vi "MainLoop2.vi"() -> ()   [LabVIEW 2021] (continued)
                                                                                                                                                                                   256705543", "Inter-pellet_interval", "0", "201", "0", "0", "0"], ["15/06/2022", "17:54:17", "                                                                                                                                                                                                                                                                                                                                                                                                                                                                                                                                                                                                                                                                                                                                                                                                                                                                                                                                                                                                                                                                                                                                                                                                                                                                                                                                                                                                                                                                                                                                                                                                                                                                                                                                                                                                                                                                                                                                                                                                                                                                                                                                                                                                                                                                                                                                                                                                                                                                                                                                                                                                                                                                                                                                                                                                                                                                                                                                                                                                                                                                                                                                                                                                                                                                                                                                                                                                                                                                                                                                                                                                                                                                                                                                                                                                                                                                                                                                                                                                                                                                                                                                                                                                                                                                                                                                                                                                                                                                                                                                                                                                                                                                                                                                                                                                                                                                                                                                                                                                                                                                                                                                                                                                                                                                                                                                                                                                                                                                                                                                                                                                                                                                                                                                                                                                                                                                                                                                                                                                                                                                                                                                                                                                                                                                                                                                                                                                                                                                                                                                                                                                                                                                                                                                                                                                                                                                                                                                                                                                                                                                                                                                                                                                                                                                                                                                                                                                                                                                                                                                                                                                                                                                                                                                                                                                                                                                                                                                                                                                                                                                                                                                                                                                                                                                                                                                                                                                                                                                                                                                                                                                                                                                                                                                                                                                                                                                                                                                                                                                                                                                                                                                                                                                                                                                                                                                                                                                                                                                                                                                                                                                                                                                                                                                                                                                                                                                                                                                                                                                                                                                                                                                                                                                                                                                                                                                                                                                                                                                                                                                                                                                                                                                                                                                                                                                                                                                                                                                                                                                                                                                                                                                                                                                                                                                                                                                                                                                                                                                                                                                                                                                                                          256715699", "3 pellets delivered total", "0", "201", "0", "0", "0"], ["15/06/2022", "17:54:17", "                                                                                                                                                                                                                                                                                                                                                                                                                                                                                                                                                                                                                                                                                                                                                                                                                                                                                                                                                                                                                                                                                                                                                                                                                                                                                                                                                                                                                                                                                                                                                                                                                                                                                                                                                                                                                                                                                                                                                                                                                                                                                                                                                                                                                                                                                                                                                                                                                                                                                                                                                                                                                                                                                                                                                                                                                                                                                                                                                                                                                                                                                                                                                                                                                                                                                                                                                                                                                                                                                                                                                                                                                                                                                                                                                                                                                                                                                                                                                                                                                                                                                                                                                                                                                                                                                                                                                                                                                                                                                                                                                                                                                                                                                                                                                                                                                                                                                                                                                                                                                                                                                                                                                                                                                                                                                                                                                                                                                                                                                                                                                                                                                                                                                                                                                                                                                                                                                                                                                                                                                                                                                                                                                                                                                                                                                                                                                                                                                                                                                                                                                                                                                                                                                                                                                                                                                                                                                                                                                                                                                                                                                                                                                                                                                                                                                                                                                                                                                                                                                                                                                                                                                                                                                                                                                                                                                                                                                                                                                                                                                                                                                                                                                                                                                                                                                                                                                                                                                                                                                                                                                                                                                                                                                                                                                                                                                                                                                                                                                                                                                                                                                                                                                                                                                                                                                                                                                                                                                                                                                                                                                                                                                                                                                                                                                                                                                                                                                                                                                                                                                                                                                                                                                                                                                                                                                                                                                                                                                                                                                                                                                                                                                                                                                                                                                                                                                                                                                                                                                                                                                                                                                                                                                                                                                                                                                                                                                                                                                                                                                                                                                                                                                                                                                                                                                                                                                                                                                                                                                                                                                                                                                                                              256716167", "3 pellets delivered total", "0", "201", "3", "0", "0"], ["15/06/2022", "17:54:50", "256749394", "3 pellets delivered total", "0", "120", "0", "0", "0"], ["15/06/2022", "17:54:50", "256749419", "Condition: j - 120", "0", "120", "0", "0", "0"], ["15/06/2022", "17:54:52", "256750710", "Nest beam break", "0", "120", "0", "0", "0"], ["15/06/2022", "18:19:22", "                                                                                                                                                                                                                                                                                                                                                                                                                                                                                                                                                                                                                                                                                                                                                                                                                                                                                                                                                                                                                                                                                                                                                                                                                                                                                                                                                                                                                                                                                                                                                                                                                                                                                                                                                                                                                                                                                                                                                                                                                                                                                                                                                                                                                                                                                                                                                                                                                                                                                                                                                                                                                                                                                                                                                                                                                                                                                                                                                                                                                                                                                                                                                                                                                                                                                                                                                                                                                                                                                                                                                                                                                                                                                                                                                                                                                                                                                                                                                                                                                                                                                                                                                                                                                                                                                                                                                                                                                                                                                                                                                                                                                                                                                                                                                                                                                                                                                                                                                                                                                                                                                                                                                                                                                                                                                                                                                                                                                                                                                                                                                                                                                                                                                                                                                                                                                                                                                                                                                                                                                                                                                                                                                                                                                                                                                                                                                                                                                                                                                                                                                                                                                                                                                                                                                                                                                                                                                                                                                                                                                                                                                                                                                                                                                                                                                                                                                                                                                                                                                                                                                                                                                                                                                                                                                                                                                                                                                                                                                                                                                                                                                                                                                                                                                                                                                                                                                                                                                                                                                                                                                                                                                                                                                                                                                                                                                                                                                                                                                                                                                                                                                                                                                                                                                                                                                                                                                                                                                                                                                                                                                                                                                                                                                                                                                                                                                                                                                                                                                                                              258221447", "1469059 ms in nest", "1469059", "120", "0", "0", "0"]]
  in  "Save event file?":bool=TRUE
  in  "file path (dialog if empty)":path=path "C:/Data/av_maze/cohort1/mouseX_202206XXtxt"
  # "Social\n\nWater\n\nFood\n\nMiddle 1\n\nMiddle 2\n\nHome cage"
  # "Low (0)     Medium (1)    High(2)"
  # "Pellets \n\nWater drops\n\nSocial time (ms)"
  # "This should stay at 1"
  # "Social                Water                  Food               Middle            Middle 2       Home cage"
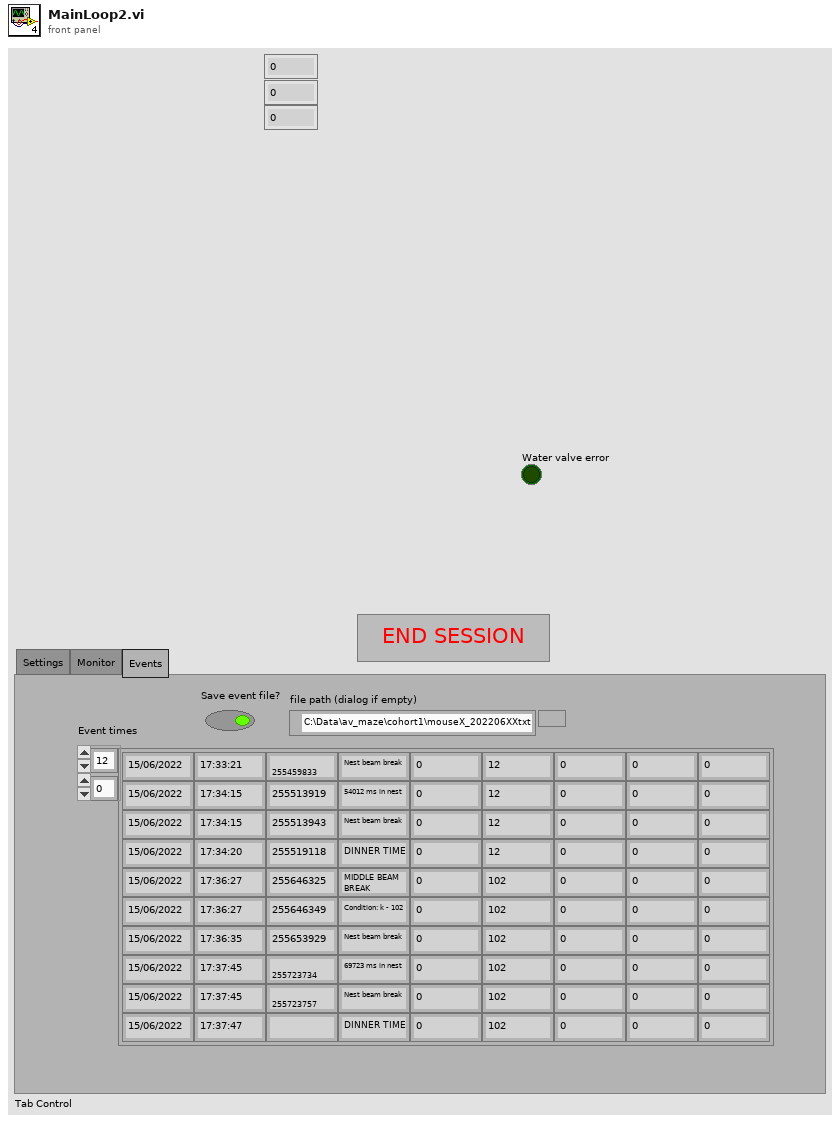
[diagram p1: front panel]
types:
  T1 = enum32{"All drives change and different", "One drive changes", "All drives same, but change"}
  T2 = typedef "XDNodeRunTimeDep.lvlib/timing_clust.ctl" = cluster{"Expected End [f-1]":u64, "Actual End [f-1]":u64, "Finished Late? [f-1]":bool, "Expected End [i-1]":u64, "Actual End [i-1]":u64, "Finished Late? [i-1]":bool, "Expected Start [i]":u64, "Actual Start [i]":u64, "Expected Start [f]":u64, "Actual Start [f]":u64, "Source Name":string, "Structure Name":string, "Period":i64, "Deadline":i64, "Offset":i64, "Start":i64, "Priority":i32, "Timeout":i32, "Mode":T3, "Wakeup Reason":T4, "Error":errorcluster, "Source Type":string, "Secondary Source Type":string, "Global End Time":u64, "Global Start Time":u64, "Frame Duration":u64, "Iteration Duration":u64, "Assigned CPU":i32, "I/O Scan Engine Mode":u32}
  T3 = typedef "XDNodeRunTimeDep.lvlib/nitl_modes.ctl" = enum32{"No Change", "Process missed periods, maintain original phase", "Discard missed periods, maintain original phase", "Process missed periods, ignore original phase", "Discard missed periods, ignore original phase"}
  T4 = typedef "XDNodeRunTimeDep.lvlib/wakeup.ctl" = enum32{"Normal", "Aborted", "Asynchronous wakeup", "Timing source error", "Timed loop error", "Timeout"}
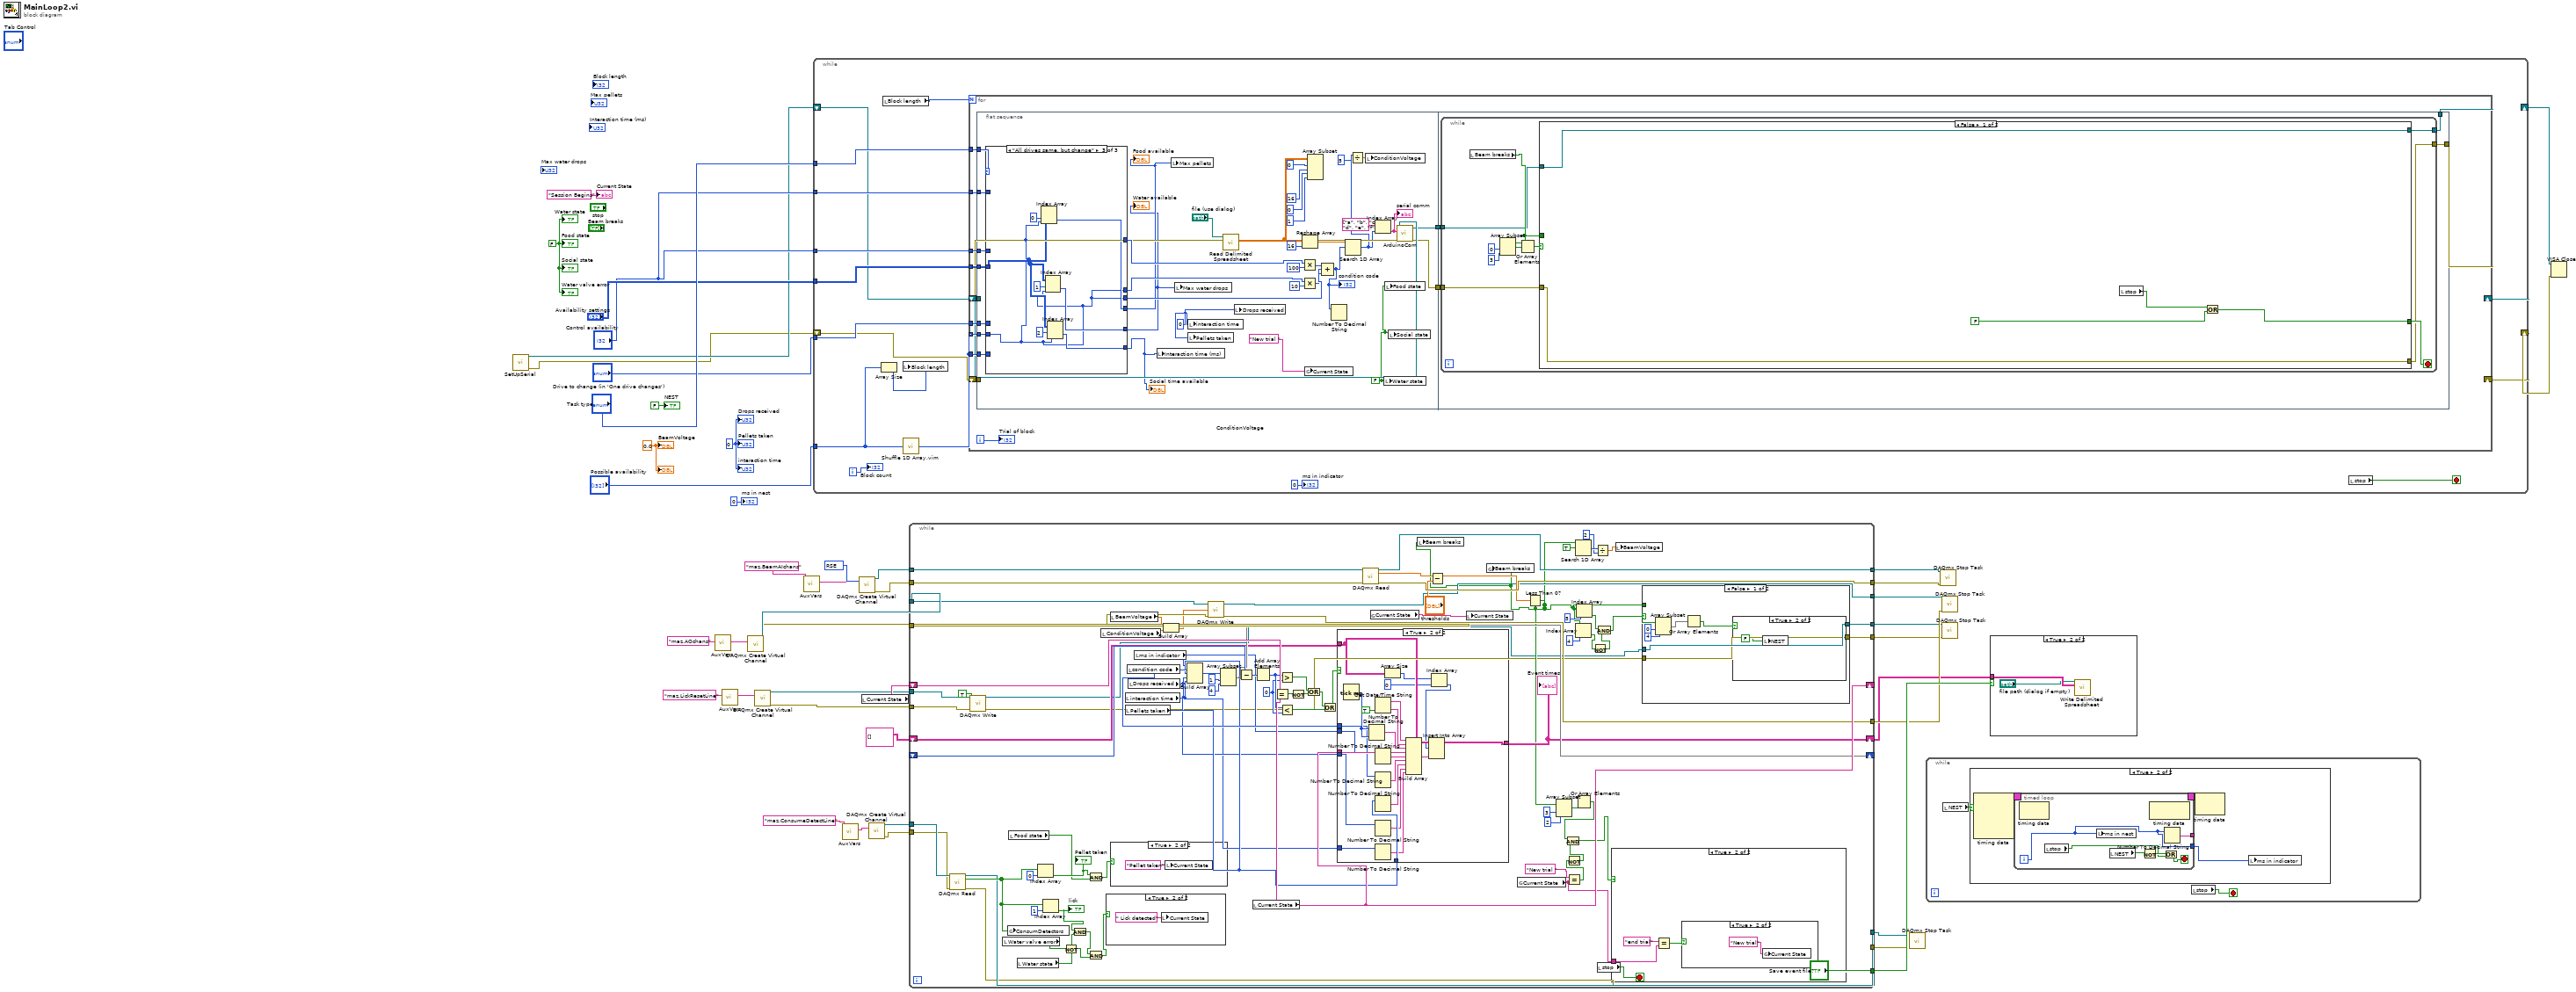
[diagram p0: block diagram]
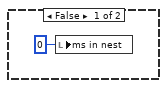
[diagram p2: hidden frame]
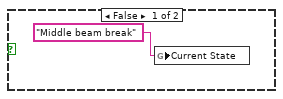
[diagram p7: hidden frame]
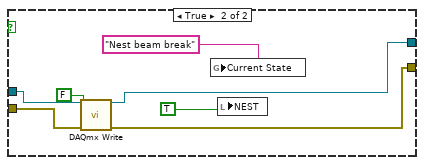
[diagram p9: hidden frame]
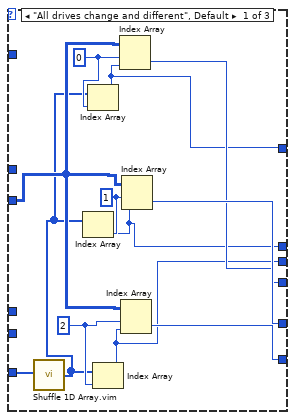
[diagram p11: hidden frame]
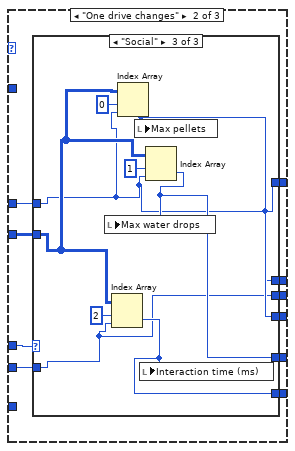
[diagram p12: hidden frame]
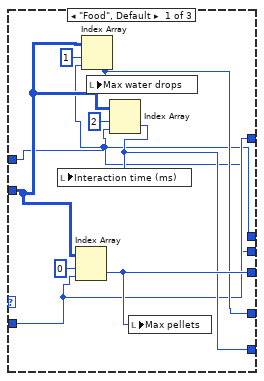
[diagram p13: hidden frame]
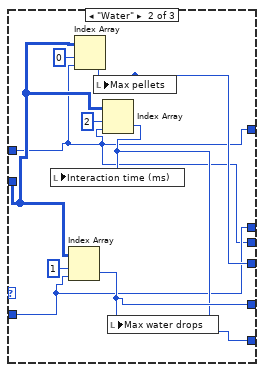
[diagram p14: hidden frame]
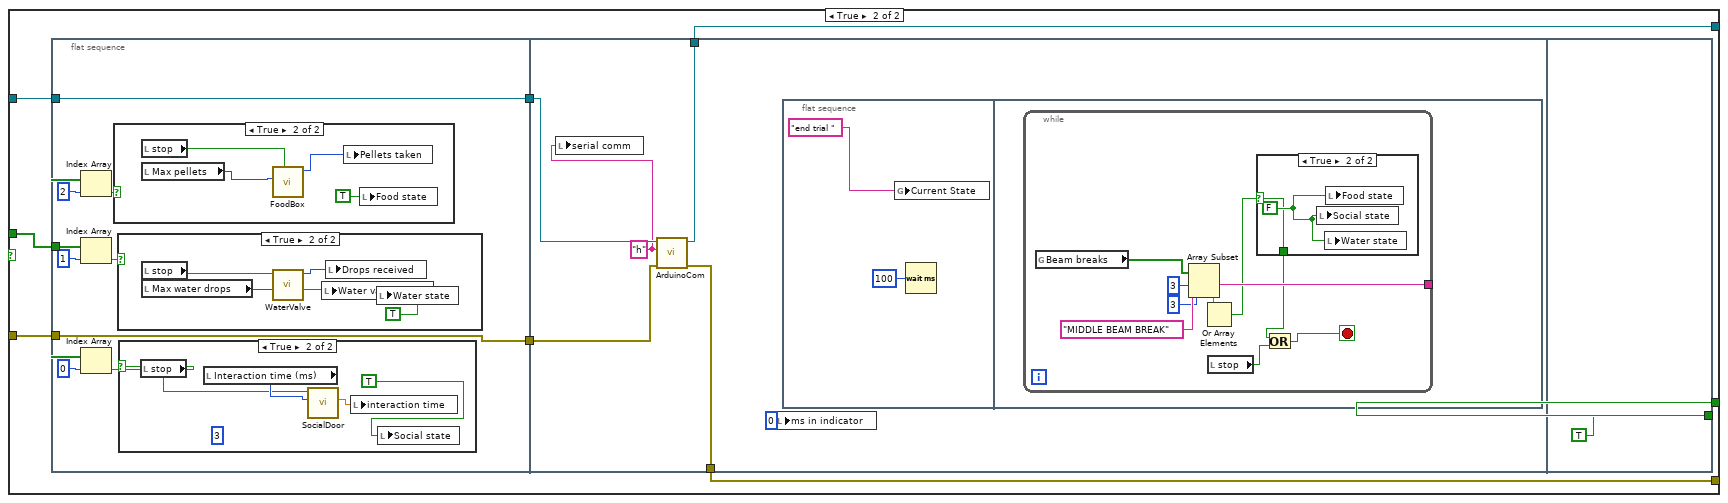
[diagram p15: hidden frame]
diagram:
  w7 = FALSE ("Water state")
  w16 = u32 0 ("Pellets taken")
  w27 = 0.0 ("BeamVoltage")
  w32 = 10083 items=["Default"=-1, "RSE"=10083, "NRSE"=10078, "Differential"=10106, "Pseudodifferential"=12529] ("input terminal configuration")
  n1 = call "SetUpSerial.vi"() -> ("error out"=w19:errorcluster, "VISA resource name out"=w34:refnum<visa-resource-name>)  [unwired: 10 in]
  n2 = call "AuxVars.vi"("key"="maz.AOchans") -> ("value"=w23:string)  [unwired: 9 in, 1 out]
  n3 = call "AuxVars.vi"("key"="maz.LickResetLine") -> ("value"=w6:string)  [unwired: 9 in, 1 out]
  n4 = call-poly <vilib>:"DAQmx Create Virtual Channel.vi"("physical channels"=w23) -> ("task out"=w29:refnum<k21>, "error out"=w28:errorcluster)  [unwired: 13 in]
  n5 = call-poly <vilib>:"DAQmx Create Virtual Channel.vi"("lines"=w6) -> ("task out"=w4:refnum<k21>, "error out"=w3:errorcluster)  [unwired: 13 in]
  n6 = call "AuxVars.vi"("key"="maz.BeamAIchans") -> ("value"=w21:string)  [unwired: 9 in, 1 out]
  n7 = while {
    tunnel: "Task type" -> [w60]
    tunnel: "Drive to change (in 'One drive changes')" -> [w59]
    tunnel: "Possible availability" -> [w54]
    tunnel: "Availability settings" -> [w58]
    tunnel: "Control availability" -> [w57]
    tunnel: "Control availability" -> [w56]
    shift-right: [w47] -> w20
    shift-left: w34 -> [w49]
    shift-right: [w46] -> w33
    shift-left: w19 -> [w48]
    i -> [w52]
    stop <- w50 stop-if-true
    n8 = Array Size(array=w54) -> (size(s)=w53:i32)
    n9 = local read "Block length"() -> (w55:i32)
    n10 = local write "Block length"(w53) -> ()
    n11 = call "Shuffle 1D Array.vim"("array"=w54) -> ("shuffled array"=w51:i32[])  [unwired: 4 in]
    n12 = for {
      N: w55 -> [_]
      tunnel: w60 -> [w74]
      tunnel: w59 -> [w73]
      tunnel: w51 -> [w72] mode=indexing
      tunnel: w58 -> [w71]
      tunnel: w57 -> [w70]
      tunnel: w56 -> [w69]
      tunnel: w51 -> [w67]
      shift-right: [w62] -> w47
      shift-left: w49 -> [w66]
      shift-right: [w61] -> w46
      shift-left: w48 -> [w65]
      i -> [w68]
      n13 = flat-sequence {
        tunnel: w74 -> [w112]
        tunnel: w73 -> [w111]
        tunnel: w72 -> [w110]
        tunnel: w71 -> [w109]
        tunnel: w70 -> [w108]
        tunnel: w69 -> [w107]
        tunnel: w67 -> [w106]
        tunnel: w66 -> [w87]
        tunnel: w65 -> [w86]
        tunnel: [w76] -> w64
        tunnel: [w75] -> w63
        tunnel: w64 -> [w173]
        tunnel: w63 -> [w172]
        tunnel: [w171] -> w62
        tunnel: [w170] -> w61
        frame #0 {
          w78 = FALSE ("Social state")
          w79 = u32 0 ("interaction time")
          n14 = case shown="\"All drives same, but change\"" w112 {
            tunnel: w111 -> [_ w134 _]
            tunnel: w110 -> [_ w133 w162]
            tunnel: w109 -> [w124 w132 w166]
            tunnel: w108 -> [_ _ _]
            tunnel: w107 -> [_ w131 _]
            tunnel: [w116 w130 w165] -> w84
            tunnel: [w117 w129 w164] -> w83
            tunnel: [w121 w128 w163] -> w85
            tunnel: w106 -> [w123 _ _]
            tunnel: [w115 w127 w162] -> w103
            tunnel: [w114 w126 w162] -> w102
            tunnel: [w113 w125 w162] -> w101
            frame "All drives change and different", Default {
              w120 = 0 ("index")
              w119 = 1 ("index")
              w122 = 2 ("index")
              n15 = call "Shuffle 1D Array.vim"("array"=w123) -> ("shuffled array"=w118:i32[])  [unwired: 4 in]
              n16 = Index Array(array=w118, index=w119) -> (element=w114:i32)
              n17 = Index Array(array=w118, index=w120) -> (element=w115:i32)
              n18 = Index Array(array=w118, index=w122) -> (element=w113:i32)
              n19 = Index Array(array=w124, index (row)=w120, index (col)=w115) -> (element=w116:i32)
              n20 = Index Array(array=w124, index (row)=w122, index (col)=w113) -> (element=w121:i32)
              n21 = Index Array(array=w124, index (row)=w119, index (col)=w114) -> (element=w117:i32)
            }
            frame "One drive changes" {
              n22 = case shown="\"Social\"" w134 {
                tunnel: w133 -> [w136 w145 w153]
                tunnel: w132 -> [w140 w149 w158]
                tunnel: w131 -> [w135 w144 w154]
                tunnel: [w139 w148 w155] -> w130
                tunnel: [w138 w147 w157] -> w129
                tunnel: [w137 w146 w156] -> w128
                tunnel: [w136 w144 w154] -> w127
                tunnel: [w135 w145 w154] -> w126
                tunnel: [w135 w144 w153] -> w125
                frame "Food", Default {
                  n23 = Index Array(array=w140, index (row)=0 ("index"), index (col)=w136) -> (element=w139:i32)
                  n24 = Index Array(array=w140, index (row)=1, index (col)=w135) -> (element=w138:i32)
                  n25 = local write "Max water drops"(w138) -> ()
                  n26 = Index Array(array=w140, index (row)=2 ("disabled index (row)"), index (col)=w135) -> (element=w137:i32)
                  n27 = local write "Interaction time (ms)"(w137) -> ()
                  n28 = local write "Max pellets"(w139) -> ()
                }
                frame "Water" {
                  n29 = Index Array(array=w149, index (row)=1 ("index"), index (col)=w145) -> (element=w147:i32)
                  n30 = Index Array(array=w149, index (row)=0, index (col)=w144) -> (element=w148:i32)
                  n31 = local write "Max pellets"(w148) -> ()
                  n32 = Index Array(array=w149, index (row)=2 ("disabled index (row)"), index (col)=w144) -> (element=w146:i32)
                  n33 = local write "Interaction time (ms)"(w146) -> ()
                  n34 = local write "Max water drops"(w147) -> ()
                }
                frame "Social" {
                  n35 = Index Array(array=w158, index (row)=2 ("index"), index (col)=w153) -> (element=w156:i32)
                  n36 = Index Array(array=w158, index (row)=0, index (col)=w154) -> (element=w155:i32)
                  n37 = local write "Max pellets"(w155) -> ()
                  n38 = local write "Interaction time (ms)"(w156) -> ()
                  n39 = Index Array(array=w158, index (row)=1 ("disabled index (row)"), index (col)=w154) -> (element=w157:i32)
                  n40 = local write "Max water drops"(w157) -> ()
                }
              }
            }
            frame "All drives same, but change" {
              n41 = Index Array(array=w166, index (row)=0, index (col)=w162) -> (element=w165:i32)
              n42 = Index Array(array=w166, index (row)=1, index (col)=w162) -> (element=w164:i32)
              n43 = Index Array(array=w166, index (row)=2, index (col)=w162) -> (element=w163:i32)
            }
          }
          "Food available" <- w84
          "Water available" <- w83
          "Social time available" <- w85
          n44 = local write "Interaction time (ms)"(w85) -> ()
          n45 = local write "Max pellets"(w84) -> ()
          n46 = local write "Max water drops"(w83) -> ()
          n47 = local write "interaction time"(w79) -> ()
          n48 = local write "Pellets taken"(w79) -> ()
          n49 = call-poly <vilib>:"Read Delimited Spreadsheet.vi"("file path (dialog if empty)"="file (use dialog)") -> ("all rows"=w93:dbl[][])  [unwired: 9 in, 5 out]
          n50 = local write "Drops received"(w79) -> ()
          n51 = Reshape Array(w93, 16 ("dimension size")) -> (w92:dbl[])
          n52 = Multiply(x=w103, y=100) -> (x*y=w99:i32)
          n53 = Multiply(x=w102, y=10) -> (x*y=w100:i32)
          n54 = global write "GlobalSTATE.vi" "Current State"("New trial " ("string")) -> ()
          n55 = Array Subset(array=w93, index (row)=0 ("index"), length (row)=16 ("length"), index (col)=0 ("index"), length (col)=1 ("length")) -> ()  [unwired: 1 out]
          n56 = Compound Arithmetic op=ADD(w99, w100, w101) -> (w88:i32)
          "condition code" <- w88
          n57 = Number To Decimal String(number=w88) -> ()  [unwired: 1 in, 1 out]
          n58 = Search 1D Array(1D array=w92, element=w88) -> (index of element=w81:i32)  [unwired: 1 in]
          n59 = Divide(x=w81, y=5) -> (x/y=w82:dbl)
          n60 = local write "ConditionVoltage"(w82) -> ()
          n61 = Index Array(array=string[] ["a", "b", "c", "d", "e", "f", "g", "h", "i", "j", "k", "l", "m", "n", "o"], index=w81) -> (element=w89:string)
          "serial comm" <- w89
          n62 = local write "Water state"(w78) -> ()
          n63 = local write "Food state"(w78) -> ()
          n64 = local write "Social state"(w78) -> ()
          n65 = call "ArduinoCom.vi"("error out"=w86, "write buffer"=w89, "VISA resource name out"=w87) -> ("error out 2"=w75:errorcluster, "VISA resource name out 2"=w76:refnum<visa-resource-name>)  [unwired: 7 in]
        }
        frame #1 {
          n66 = while {
            tunnel: w173 -> [w177]
            tunnel: w172 -> [w176]
            tunnel: [w175] -> w171
            tunnel: [w174] -> w170
            stop <- w178 stop-if-true
            n67 = local read "Beam breaks"() -> (w179:bool[])
            n68 = Array Subset(array=w179, index=0, length=3) -> (w182:bool[])
            n69 = Or Array Elements(Boolean array=w182) -> (logical OR=w183:bool)
            n70 = case shown="False" w183 {
              tunnel: w179 -> [_ w196]
              tunnel: [w186 w195] -> w178
              tunnel: w177 -> [w185 w193]
              tunnel: w176 -> [w184 w191]
              tunnel: [w185 w190] -> w175
              tunnel: [w184 w189] -> w174
              frame False {
                n71 = local read "stop"() -> (w187:bool)
                n72 = Or(x=w187, y=FALSE ("stop")) -> (x .or. y?=w186:bool)
              }
              frame True {
                n73 = flat-sequence {
                  tunnel: w196 -> [w199]
                  tunnel: [w198] -> w194
                  tunnel: w193 -> [w198]
                  tunnel: [w197] -> w192
                  tunnel: w191 -> [w197]
                  tunnel: w194 -> [w223]
                  tunnel: w192 -> [w222]
                  tunnel: [w220] -> w190
                  tunnel: [w219] -> w189
                  tunnel: [TRUE ("stop")] -> w195
                  frame #0 {
                    n74 = Index Array(array=w199, index=2) -> (element=w204:bool)
                    n75 = Index Array(array=w199, index=1) -> (element=w200:bool)
                    n76 = Index Array(array=w199, index=0) -> (element=w202:bool)
                    n77 = case shown="True" w204 {
                      frame False {
                      }
                      frame True {
                        n78 = local read "stop"() -> (w217:bool)
                        n79 = local read "Max pellets"() -> (w218:u32)
                        n80 = call "FoodBox.vi"("STOP"=w217, "Max pellets"=w218) -> ("Pellets taken"=w216:i32)  [unwired: 8 in, 1 out]
                        n81 = local write "Pellets taken"(w216) -> ()
                        n82 = local write "Food state"(TRUE ("Food state")) -> ()
                      }
                    }
                    n83 = case shown="True" w200 {
                      frame False {
                      }
                      frame True {
                        n84 = local read "stop"() -> (w209:bool)
                        n85 = local read "Max water drops"() -> (w210:u32)
                        n86 = call "WaterValve.vi"("Max pulses"=w210, "STOP"=w209) -> ("Error"=w206:bool, "Number pulses"=w208:u32)  [unwired: 8 in]
                        n87 = local write "Water valve error"(w206) -> ()
                        n88 = local write "Drops received"(w208) -> ()
                        n89 = local write "Water state"(TRUE ("Water state")) -> ()
                      }
                    }
                    n90 = case shown="True" w202 {
                      frame False {
                      }
                      frame True {
                        (unwired) 3 ("index")
                        n91 = local read "stop"() -> (w213:bool)
                        n92 = local read "Interaction time (ms)"() -> (w214:u32)
                        n93 = call "SocialDoor.vi"("Interaction time"=w214, "STOP"=w213) -> ("Time spent"=w212:dbl)  [unwired: 9 in]
                        n94 = local write "interaction time"(w212) -> ()
                        n95 = local write "Social state"(TRUE ("Water state")) -> ()
                      }
                    }
                  }
                  frame #1 {
                    w221 = "h" ("write buffer")
                    n96 = local write "serial comm"(w221) -> ()
                    n97 = call "ArduinoCom.vi"("error out"=w222, "write buffer"=w221, "VISA resource name out"=w223) -> ("error out 2"=w219:errorcluster, "VISA resource name out 2"=w220:refnum<visa-resource-name>)  [unwired: 7 in]
                    n98 = local write "ms in indicator"(0 ("ms in nest")) -> ()
                    n99 = flat-sequence {
                      frame #0 {
                        n100 = global write "GlobalSTATE.vi" "Current State"("end trial " ("string")) -> ()
                        n101 = Wait (ms)(milliseconds to wait=u32 100) -> ()  [unwired: 1 out]
                      }
                      frame #1 {
                        n102 = while {
                          tunnel: ["MIDDLE BEAM BREAK" ("Current State")] -> _
                          stop <- w233 stop-if-true
                          n103 = global read "Global_BeamBreaks.vi" "Beam breaks"() -> (w230:bool[])
                          n104 = Array Subset(array=w230, index=3, length=3) -> (w229:bool[])
                          n105 = Or Array Elements(Boolean array=w229) -> (logical OR=w228:bool)
                          n106 = local read "stop"() -> (w234:bool)
                          n107 = case shown="True" w228 {
                            selector: w228 -> [w236 w237]
                            tunnel: [w236 w237] -> w227
                            frame False {
                            }
                            frame True {
                              w238 = FALSE ("Social state")
                              n108 = local write "Social state"(w238) -> ()
                              n109 = local write "Water state"(w238) -> ()
                              n110 = local write "Food state"(w238) -> ()
                            }
                          }
                          n111 = Or(x=w227, y=w234) -> (x .or. y?=w233:bool)
                        }
                      }
                    }
                  }
                  frame #2 {
                  }
                }
              }
            }
          }
        }
      }
      "Trial of block" <- w68
    }
    n112 = local read "stop"() -> (w50:bool)
    "Block count" <- w52
  }
  n113 = call "AuxVars.vi"("key"="maz.ConsumeDetectLine") -> ("value"=w12:string)  [unwired: 9 in, 1 out]
  n114 = call-poly <vilib>:"DAQmx Create Virtual Channel.vi"("input terminal configuration"=w32, "physical channels"=w21) -> ("task out"=w45:refnum<k21>, "error out"=w44:errorcluster)  [unwired: 12 in]
  n115 = local read "Current State"() -> (w35:string)
  n116 = call-poly <vilib>:"DAQmx Create Virtual Channel.vi"("lines"=w12) -> ("task out"=w11:refnum<k21>, "error out"=w10:errorcluster)  [unwired: 13 in]
  n117 = while {
    tunnel: w45 -> [w322]
    tunnel: w44 -> [w321]
    tunnel: [w320] -> w43
    tunnel: [w319] -> w42
    shift-right: [w316] -> _
    shift-left: w35 -> [w315]
    tunnel: ["Save event file?"] -> w31
    tunnel: w29 -> [w308]
    tunnel: w28 -> [w307]
    tunnel: [w299] -> w26
    tunnel: [w298] -> w25
    shift-right: [w292] -> _
    shift-left: _ -> [w297]
    shift-right: [w284] -> w18
    shift-left: string[][] [] -> [w283]
    tunnel: w11 -> [w274]
    tunnel: w10 -> [w273]
    tunnel: [w267] -> w9
    tunnel: [w266] -> w8
    tunnel: w4 -> [w246]
    tunnel: w3 -> [w245]
    tunnel: [w241] -> w2
    tunnel: [w240] -> w1
    stop <- w318 stop-if-true
    w289 = u32 0 ("y")
    n118 = call-poly <vilib>:"DAQmx Read.vi"("task/channels in"=w274, "error in"=w273) -> ("task out"=w267:refnum<k21>, "data"=w270:bool[], "error out"=w266:errorcluster)  [unwired: 11 in]
    n119 = call-poly <vilib>:"DAQmx Write.vi"("task/channels in"=w246, "data"=TRUE, "error in"=w245) -> ("task out"=w243:refnum<k21>, "error out"=w242:errorcluster)  [unwired: 10 in, 1 out]
    n120 = local read "Water valve error"() -> (w262:bool)
    n121 = global write "Global_BeamBreaks.vi" "ConsumDetectors"(w270) -> ()
    n122 = local read "Food state"() -> (w263:bool)
    n123 = local read "Water state"() -> (w268:bool)
    n124 = Index Array(array=w270, index=0) -> (element=w264:bool)
    "Pellet taken" <- w264
    n125 = Index Array(array=w270, index=1) -> (element=w269:bool)
    "lick" <- w269
    n126 = Not(x=w262) -> (.not. x?=w261:bool)
    n127 = And(x=w269, y=w268) -> (x .and. y?=w260:bool)
    n128 = And(x=w264, y=w263) -> (x .and. y?=w265:bool)
    n129 = And(x=w260, y=w261) -> (x .and. y?=w259:bool)
    n130 = local read "ConditionVoltage"() -> (w301:dbl)
    n131 = case shown="True" w259 {
      frame False {
      }
      frame True {
        n132 = local write "Current State"(" Lick detected" ("Current State")) -> ()
      }
    }
    n133 = local read "BeamVoltage"() -> (w302:dbl)
    n134 = case shown="True" w265 {
      frame False {
      }
      frame True {
        n135 = local write "Current State"("Pellet taken" ("Current State")) -> ()
      }
    }
    n136 = local read "interaction time"() -> (w278:u32)
    n137 = local read "Pellets taken"() -> (w281:u32)
    n138 = local read "condition code"() -> (w282:i32)
    n139 = local read "Drops received"() -> (w280:u32)
    n140 = local read "ms in indicator"() -> (w279:i32)
    n141 = Build Array(w302, w301) -> (w300:dbl[])
    n142 = Build Array(w279, w282, w281, w280, w278) -> (w285:u32[])
    n143 = call-poly <vilib>:"DAQmx Write.vi"("task/channels in"=w308, "data"=w300, "error in"=w307) -> ("task out"=w299:refnum<k21>, "error out"=w298:errorcluster)  [unwired: 10 in, 1 out]
    n144 = Array Subset(array=w285, index=1, length=4) -> (w292:u32[])
    n145 = Subtract(x=w297, y=w292) -> (x-y=w291:u32[])
    n146 = local read "Current State"() -> (w316:string)
    n147 = Add Array Elements(numeric array=w291) -> (sum=w290:u32)
    n148 = Equal?(x=w315, y=w316) -> (x = y?=w317:bool)
    n149 = Greater?(x=w290, y=w289) -> (0:w295:bool)
    n150 = Less?(x=w290, y=w289) -> (x < y?=w287:bool)
    n151 = Not(x=w317) -> (.not. x?=w296:bool)
    n152 = Or(x=w295, y=w296) -> (x .or. y?=w288:bool)
    n153 = Or(x=w288, y=w287) -> (x .or. y?=w286:bool)
    n154 = case shown="True" w286 {
      tunnel: [w345 w360] -> w284
      tunnel: w316 -> [_ w362]
      tunnel: w283 -> [w345 w359]
      tunnel: w279 -> [_ w355]
      tunnel: w282 -> [_ w353]
      tunnel: w281 -> [_ w351]
      tunnel: w280 -> [_ w349]
      tunnel: w278 -> [_ w346]
      frame False {
      }
      frame True {
        n155 = Tick Count (ms)() -> (millisecond timer value=w366:u32)
        n156 = Number To Decimal String(number=w366, width (-)=w366) -> (decimal integer string=w363:string)
        n157 = Get Date/Time String(want seconds? (F)=TRUE) -> (date string=w365:string, time string=w364:string)  [unwired: 2 in]
        n158 = Number To Decimal String(number=w355) -> (decimal integer string=w354:string)  [unwired: 1 in]
        n159 = Number To Decimal String(number=w353) -> (decimal integer string=w352:string)  [unwired: 1 in]
        n160 = Number To Decimal String(number=w351) -> (decimal integer string=w350:string)  [unwired: 1 in]
        n161 = Number To Decimal String(number=w349) -> (decimal integer string=w348:string)  [unwired: 1 in]
        n162 = Number To Decimal String(number=w346) -> (decimal integer string=w347:string)  [unwired: 1 in]
        n163 = Array Size(array=w359) -> (size(s)=w358:i32[])
        n164 = Build Array(w365, w364, w363, w362, w354, w352, w350, w348, w347) -> (w361:string[])
        n165 = Index Array(array=w358, index=0) -> (element=w356:i32)
        n166 = Insert Into Array(array=w359, index (row)=w356, new element=w361) -> (w360:string[][])  [unwired: 1 in]
      }
    }
    "Event times" <- w284
    n167 = call-poly <vilib>:"DAQmx Read.vi"("task/channels in"=w322, "error in"=w321) -> ("task out"=w320:refnum<k21>, "data"=w312:dbl[], "error out"=w319:errorcluster)  [unwired: 11 in]
    n168 = global read "GlobalSTATE.vi" "Current State"() -> (w314:string)
    n169 = Subtract(x=w312, y="thresholds") -> (x-y=w313:dbl[])
    n170 = local write "Current State"(w314) -> ()
    n171 = global read "GlobalSTATE.vi" "Current State"() -> (w247:string)
    n172 = Less Than 0?(x=w313) -> (x < 0?=w257:bool[])
    n173 = local write "Beam breaks"(w257) -> ()
    n174 = global write "Global_BeamBreaks.vi" "Beam breaks"(w257) -> ()
    n175 = Array Subset(array=w257, index=3, length=2) -> (w275:bool[])
    n176 = Equal?(x="New trial " ("string"), y=w247) -> (x = y?=w251:bool)
    n177 = Not(x=w251) -> (.not. x?=w252:bool)
    n178 = Search 1D Array(1D array=w257, element=TRUE) -> (index of element=w306:i32)  [unwired: 1 in]
    n179 = Index Array(array=w257, index=4) -> (element=w256:bool)
    n180 = Or Array Elements(Boolean array=w275) -> (logical OR=w249:bool)
    n181 = And(x=w249, y=w252) -> (x .and. y?=w248:bool)
    n182 = Index Array(array=w257, index=5) -> (element=w254:bool)
    n183 = Not(x=w256) -> (.not. x?=w255:bool)
    n184 = Divide(x=w306, y=2) -> (x/y=w304:dbl)
    n185 = And(x=w254, y=w255) -> (x .and. y?=w253:bool)
    n186 = local read "stop"() -> (w318:bool)
    n187 = case shown="True" w248 {
      tunnel: w247 -> [_ w326]
      frame False {
      }
      frame True {
        n188 = Equal?(x="end trial" ("string"), y=w326) -> (x = y?=w325:bool)
        n189 = case shown="True" w325 {
          frame False {
            n190 = global write "GlobalSTATE.vi" "Current State"("Middle beam break" ("Current State")) -> ()
          }
          frame True {
            n191 = global write "GlobalSTATE.vi" "Current State"("New trial" ("Current State")) -> ()
          }
        }
      }
    }
    n192 = local write "BeamVoltage"(w304) -> ()
    n193 = case shown="False" w253 {
      tunnel: w257 -> [w336 _]
      tunnel: w243 -> [w331 w342]
      tunnel: w242 -> [w330 w341]
      tunnel: [w331 w339] -> w241
      tunnel: [w330 w338] -> w240
      frame False {
        n194 = Array Subset(array=w336, index=0, length=4) -> (w333:bool[])
        n195 = Or Array Elements(Boolean array=w333) -> (logical OR=w332:bool)
        n196 = case shown="True" w332 {
          frame False {
          }
          frame True {
            n197 = local write "NEST"(FALSE) -> ()
          }
        }
      }
      frame True {
        n198 = call-poly <vilib>:"DAQmx Write.vi"("task/channels in"=w342, "data"=FALSE, "error in"=w341) -> ("task out"=w339:refnum<k21>, "error out"=w338:errorcluster)  [unwired: 10 in, 1 out]
        n199 = global write "GlobalSTATE.vi" "Current State"("Nest beam break" ("Current State")) -> ()
        n200 = local write "NEST"(TRUE) -> ()
      }
    }
  }
  n201 = call <vilib>:"DAQmx Stop Task.vi"("task/channels in"=w9, "error in"=w8) -> ()  [unwired: 12 in, 2 out]
  n202 = while {
    stop <- w368 stop-if-true
    n203 = local read "NEST"() -> (w369:bool)
    n204 = case shown="True" w369 {
      frame False {
        n205 = local write "ms in nest"(0 ("ms in nest")) -> ()
      }
      frame True {
        n206 = node-c288() -> (w373:T2)  [unwired: 4 in]
        n207 = timed-loop {
          timing: w373 -> [_]
          timing-out: [_] -> w372
          tunnel: [w378] -> _
          tunnel: [w374] -> w371
          i -> [w374]
          stop <- w375 stop-if-true
          n208 = node-c288() -> ()  [unwired: 1 in, 1 out]
          n209 = local read "stop"() -> (w376:bool)
          n210 = local write "ms in nest"(w374) -> ()
          n211 = local read "NEST"() -> (w379:bool)
          n212 = Not(x=w379) -> (.not. x?=w377:bool)
          n213 = node-c288() -> ()  [unwired: 1 in, 1 out]
          n214 = Or(x=w377, y=w376) -> (x .or. y?=w375:bool)
          n215 = Number To Decimal String(number=w374) -> (decimal integer string=w378:string)  [unwired: 1 in]
        }
        n216 = node-c288(w372) -> ()  [unwired: 1 out]
        n217 = local write "ms in indicator"(w371) -> ()
      }
    }
    n218 = local read "stop"() -> (w368:bool)
  }
  n219 = call <vilib>:"DAQmx Stop Task.vi"("task/channels in"=w43, "error in"=w42) -> ()  [unwired: 12 in, 2 out]
  n220 = call <vilib>:"DAQmx Stop Task.vi"("task/channels in"=w26, "error in"=w25) -> ()  [unwired: 12 in, 2 out]
  n221 = call <vilib>:"DAQmx Stop Task.vi"("task/channels in"=w2, "error in"=w1) -> ()  [unwired: 12 in, 2 out]
  n222 = case shown="True" w31 {
    tunnel: w18 -> [_ w385]
    frame False {
    }
    frame True {
      n223 = call-poly <vilib>:"Write Delimited Spreadsheet.vi"("file path (dialog if empty)"="file path (dialog if empty)", "2D data"=w385) -> ()  [unwired: 12 in, 2 out]
    }
  }
  n224 = VISA Close(VISA resource name=w20, error in (no error)=w33) -> ()  [unwired: 1 out]
  "Current State" <- "Session Begins" ("Current State")
  "ms in nest" <- 0 ("ms in nest")
  "NEST" <- FALSE ("NEST")
  "BeamVoltage" <- w27
  "ConditionVoltage" <- w27
  "interaction time" <- w16
  "Drops received" <- w16
  "Pellets taken" <- w16
  "ms in indicator" <- 0 ("ms in indicator")
  "Food state" <- w7
  "Social state" <- w7
  "Water state" <- w7
  "Water valve error" <- w7
